vi "Create Variable Name Array.vi"(8 "Error In":errorcluster, 9 "Name Root":string="X", 10 "First Index":i32=1, 11 "# Variables":i32) -> (0 "Error Out":errorcluster, 3 "Variable Names":string[](array[string]))   [LabVIEW 2021, in "Formula.lvlib"]
uses:
  Formula.lvlib
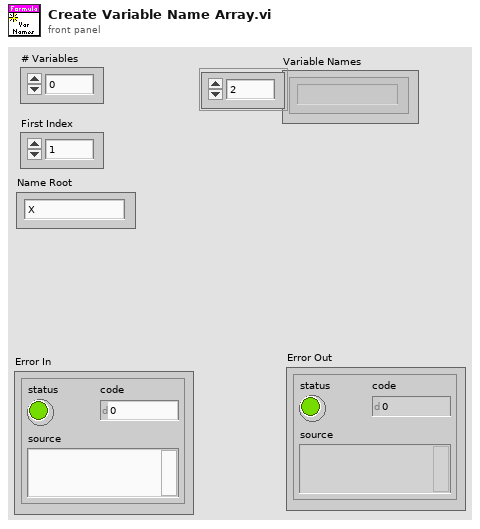
[diagram p1: front panel]
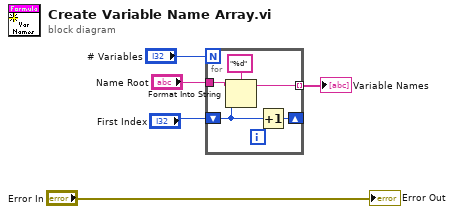
[diagram p0: block diagram]
diagram:
  n1 = for {
    N: "# Variables" -> [_]
    tunnel: "Name Root" -> [w10]
    shift-right: [w7] -> _
    shift-left: "First Index" -> [w8]
    tunnel: [w6] -> w1 mode=indexing
    n2 = Format Into String(format string="%d", initial string=w10, w8) -> (resulting string=w6:string)  [unwired: 1 in, 1 out]
    n3 = Increment(x=w8) -> (x+1=w7:i32)
  }
  "Variable Names" <- w1
  "Error Out" <- "Error In"
